vi "hydrolysis_reactor_setup.vi"(10 "#":i32) -> (2 "spec_file":path)   [LabVIEW 2019]
uses:
  lib/libSimulationControl/libSimulationControl.lvlib
  lib/libCheckpointUpdate/libCheckpointUpdate.lvlib
  lib/libFileFunctions/libFileFunctions.lvlib
panel:
  out "inflow path":path
  # "*******************************************************************\nBiogas Plant Control\n\nAuthor: Paul Zügel\nGCSC-Frankfurt am Main 2020\n\n*******************************************************************"
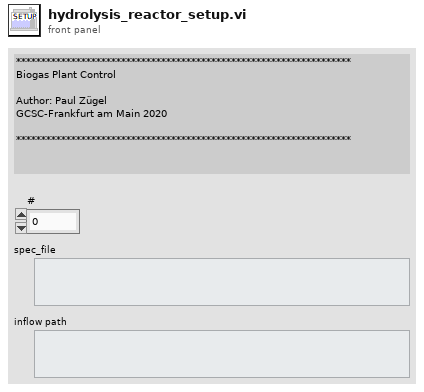
[diagram p1: front panel]
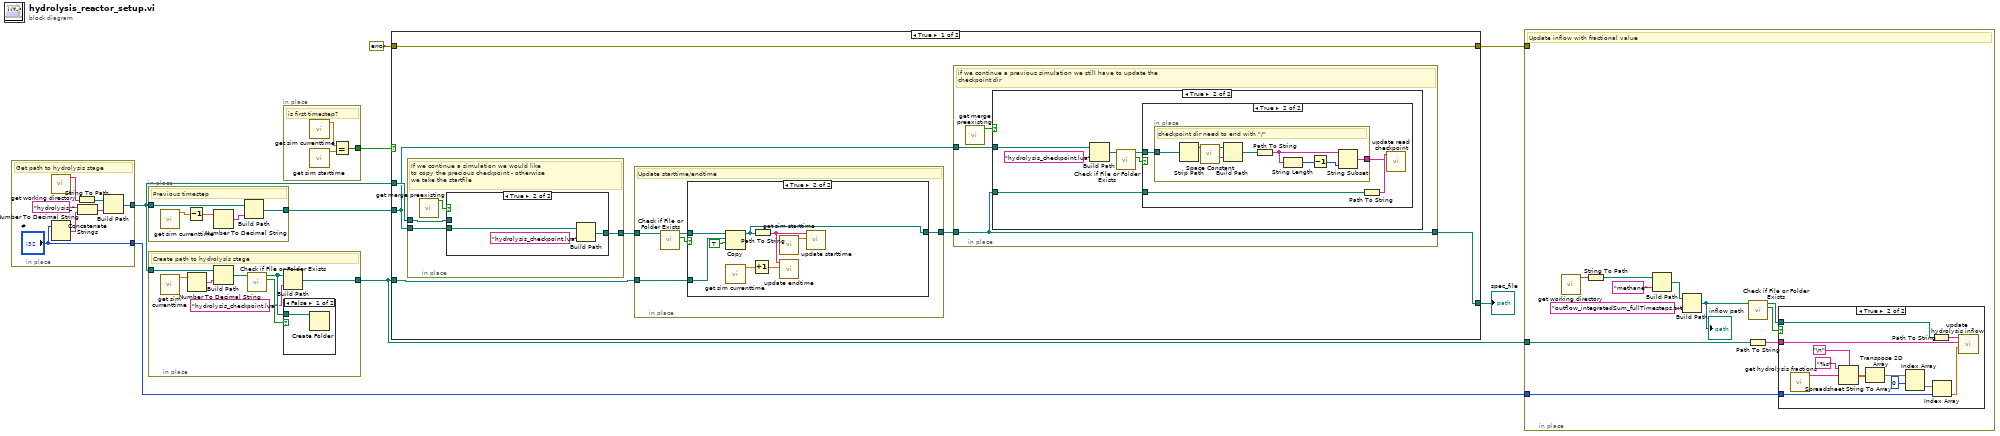
[diagram p0: block diagram]
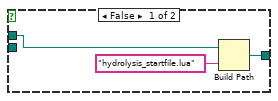
[diagram p4: hidden frame]
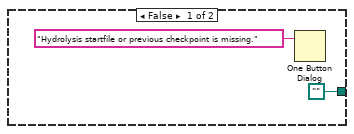
[diagram p5: hidden frame]
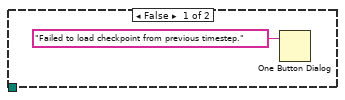
[diagram p7: hidden frame]
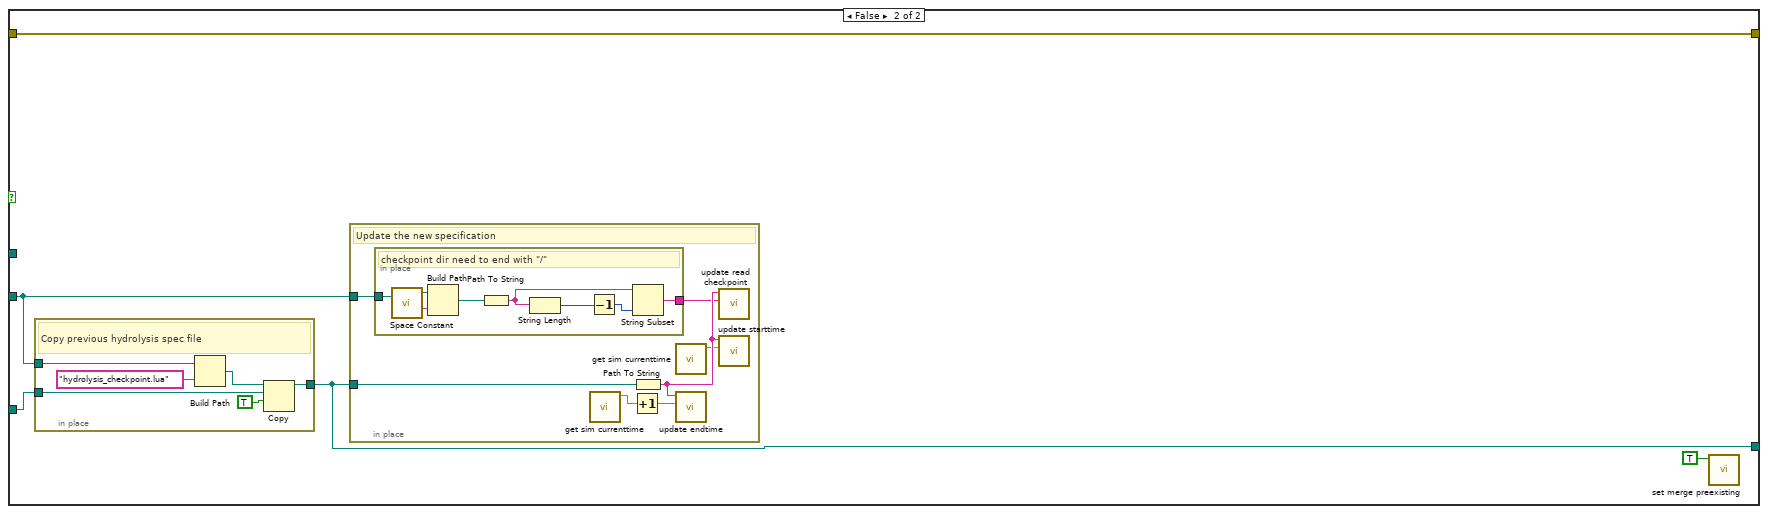
[diagram p8: hidden frame]
diagram:
  n1 = in-place {
    in-place-border: [w10] -> w4
    in-place-border: ["#"] -> w3
    # "Get path to hydrolysis stage"
    n2 = call "get working directory.vi"() -> ("function return"=w14:string)  [unwired: 10 in, 1 out]
    n3 = Number To Decimal String(number="#") -> (decimal integer string=w15:string)  [unwired: 1 in]
    n4 = String To Path(string=w14) -> (path=w11:path)
    n5 = Concatenate Strings("hydrolysis_" ("string"), w15) -> (w13:string)
    n6 = Build Path(base path=w11, name or relative path=w13) -> (appended path=w10:path)
  }
  n7 = in-place {
    in-place-border: [w18] -> w5
    in-place-border: w4 -> [w16]
    # "Previous timestep"
    n8 = call "get sim currenttime.vi"() -> ("current_time"=w17:dbl)  [unwired: 10 in, 1 out]
    n9 = Decrement(x=w17) -> (x-1=w20:dbl)
    n10 = Number To Decimal String(number=w20) -> (decimal integer string=w19:string)  [unwired: 1 in]
    n11 = Build Path(base path=w16, name or relative path=w19) -> (appended path=w18:path)
  }
  n12 = in-place {
    in-place-border: [w23] -> w7
    in-place-border: w4 -> [w21]
    # "Create path to hydrolysis stage"
    n13 = call "get sim currenttime.vi"() -> ("current_time"=w22:dbl)  [unwired: 10 in, 1 out]
    n14 = Number To Decimal String(number=w22) -> (decimal integer string=w27:string)  [unwired: 1 in]
    n15 = Build Path(base path=w21, name or relative path=w27) -> (appended path=w26:path)
    n16 = call <vilib>:"Check if File or Folder Exists.vi"("path"=w26) -> ("file or folder exists?"=w28:bool, "dup path"=w25:path)  [unwired: 8 in, 1 out]
    n17 = Build Path(base path=w25, name or relative path="hydrolysis_checkpoint.lua" ("string")) -> (appended path=w23:path)
    n18 = case shown="False" w28 {
      tunnel: w25 -> [w29 _]
      frame False {
        n19 = Create Folder(path (use dialog)=w29) -> ()  [unwired: 2 in, 3 out]
      }
      frame True {
      }
    }
  }
  n20 = in-place {
    in-place-border: [w32] -> w8
    # "is first timestep?"
    n21 = call "get sim currenttime.vi"() -> ("current_time"=w30:dbl)  [unwired: 10 in, 1 out]
    n22 = call "get sim starttime.vi"() -> ("sim_starttime"=w31:dbl)  [unwired: 10 in, 1 out]
    n23 = Equal?(x=w30, y=w31) -> (x = y?=w32:bool)
  }
  n24 = case shown="True" w8 {
    tunnel: w7 -> [w35 w89]
    tunnel: [w39 w91] -> w6
    tunnel: w5 -> [w36 w90]
    tunnel: w4 -> [w37 _]
    tunnel: errorcluster {"status"=FALSE, "code"=0, "source"=""} ("error constant") -> [w33 w87]
    tunnel: [w33 w87] -> w1
    frame True {
      n25 = in-place {
        in-place-border: [w43] -> w38
        in-place-border: w37 -> [w41]
        in-place-border: w36 -> [w40]
        # "If we continue a simulation we would like\nto copy the precious checkpoint - otherwise\nwe take the startfile"
        n26 = call "get merge preexisting.vi"() -> ("function return"=w42:bool)  [unwired: 10 in, 1 out]
        n27 = case shown="True" w42 {
          tunnel: [w45 w48] -> w43
          tunnel: w41 -> [w44 _]
          tunnel: w40 -> [_ w47]
          frame False {
            # "Copy base specification and update starttime/endtime"
            n28 = Build Path(base path=w44, name or relative path="hydrolysis_startfile.lua") -> (appended path=w45:path)
          }
          frame True {
            # "Copy previous hydrolysis spec file"
            n29 = Build Path(base path=w47, name or relative path="hydrolysis_checkpoint.lua" ("string")) -> (appended path=w48:path)
          }
        }
      }
      n30 = in-place {
        in-place-border: w38 -> [w52]
        in-place-border: w35 -> [w51]
        in-place-border: [w50] -> w34
        # "Update starttime/endtime"
        n31 = call <vilib>:"Check if File or Folder Exists.vi"("path"=w52) -> ("file or folder exists?"=w53:bool, "dup path"=w54:path)  [unwired: 8 in, 1 out]
        n32 = case shown="True" w53 {
          tunnel: [path "" w64] -> w50
          tunnel: w54 -> [_ w61]
          tunnel: w51 -> [_ w60]
          frame False {
            n33 = One Button Dialog(message="Hydrolysis startfile or previous checkpoint is missing.") -> ()  [unwired: 1 in, 1 out]
          }
          frame True {
            # "Update starttime/endtime"
            n34 = Copy(9:TRUE ("overwrite (F)"), 10:w60, 11:w61) -> (3:w64:path)  [unwired: 2 in, 2 out]
            n35 = call "get sim currenttime.vi"() -> ("current_time"=w59:dbl)  [unwired: 10 in, 1 out]
            n36 = Increment(x=w59) -> (x+1=w58:dbl)
            n37 = Path To String(path=w64) -> (string=w62:string)
            n38 = call "get sim starttime.vi"() -> ("sim_starttime"=w57:dbl)  [unwired: 10 in, 1 out]
            n39 = call "update endtime.vi"("endtime"=w58, "spec_dir"=w62) -> ()  [unwired: 9 in, 1 out]
            n40 = call "update starttime.vi"("starttime"=w57, "spec_dir"=w62) -> ()  [unwired: 9 in, 1 out]
          }
        }
      }
      n41 = in-place {
        in-place-border: [w65] -> w39
        in-place-border: w36 -> [w66]
        in-place-border: w34 -> [w65]
        # "if we continue a previous simulation we still have to update the \ncheckpoint dir"
        n42 = call "get merge preexisting.vi"() -> ("function return"=w67:bool)  [unwired: 10 in, 1 out]
        n43 = case shown="True" w67 {
          tunnel: w66 -> [_ w72]
          tunnel: w65 -> [_ w68]
          frame False {
          }
          frame True {
            n44 = Build Path(base path=w72, name or relative path="hydrolysis_checkpoint.lua" ("string")) -> (appended path=w71:path)
            n45 = call <vilib>:"Check if File or Folder Exists.vi"("path"=w71) -> ("file or folder exists?"=w69:bool, "dup path"=w70:path)  [unwired: 8 in, 1 out]
            n46 = case shown="True" w69 {
              tunnel: w70 -> [_ w76]
              tunnel: w68 -> [_ w77]
              frame False {
                n47 = One Button Dialog(message="Failed to load checkpoint from previous timestep.") -> ()  [unwired: 1 in, 1 out]
              }
              frame True {
                n48 = in-place {
                  in-place-border: w76 -> [w86]
                  in-place-border: [w79] -> w75
                  # "checkpoint dir need to end with \"/\""
                  n49 = Strip Path(path=w86) -> (stripped path=w80:path)  [unwired: 1 out]
                  n50 = call <vilib>:"Space Constant.vi"() -> ("String"=w81:string)
                  n51 = Build Path(base path=w80, name or relative path=w81) -> (appended path=w84:path)
                  n52 = Path To String(path=w84) -> (string=w85:string)
                  n53 = String Length(string=w85) -> (length=w83:i32)
                  n54 = Decrement(x=w83) -> (x-1=w82:i32)
                  n55 = String Subset(string=w85, length (rest)=w82) -> (substring=w79:string)  [unwired: 1 in]
                }
                n56 = Path To String(path=w77) -> (string=w78:string)
                n57 = call "update read checkpoint.vi"("checkpoint_dir"=w75, "spec_dir"=w78) -> ()  [unwired: 9 in, 1 out]
              }
            }
          }
        }
      }
    }
    frame False {
      n58 = in-place {
        in-place-border: w89 -> [w108]
        in-place-border: [w107] -> w91
        in-place-border: w90 -> [w106]
        # "Copy previous hydrolysis spec file"
        n59 = Build Path(base path=w106, name or relative path="hydrolysis_checkpoint.lua" ("string")) -> (appended path=w110:path)
        n60 = Copy(9:TRUE ("overwrite (F)"), 10:w108, 11:w110) -> (3:w107:path)  [unwired: 2 in, 2 out]
      }
      n61 = in-place {
        in-place-border: w90 -> [w92]
        in-place-border: w91 -> [w94]
        # "Update the new specification"
        n62 = in-place {
          in-place-border: [w100] -> w93
          in-place-border: w92 -> [w99]
          # "checkpoint dir need to end with \"/\""
          n63 = call <vilib>:"Space Constant.vi"() -> ("String"=w101:string)
          n64 = Build Path(base path=w99, name or relative path=w101) -> (appended path=w104:path)
          n65 = Path To String(path=w104) -> (string=w105:string)
          n66 = String Length(string=w105) -> (length=w103:i32)
          n67 = Decrement(x=w103) -> (x-1=w102:i32)
          n68 = String Subset(string=w105, length (rest)=w102) -> (substring=w100:string)  [unwired: 1 in]
        }
        n69 = call "get sim currenttime.vi"() -> ("current_time"=w96:dbl)  [unwired: 10 in, 1 out]
        n70 = Increment(x=w96) -> (x+1=w95:dbl)
        n71 = Path To String(path=w94) -> (string=w98:string)
        n72 = call "get sim currenttime.vi"() -> ("current_time"=w97:dbl)  [unwired: 10 in, 1 out]
        n73 = call "update endtime.vi"("endtime"=w95, "spec_dir"=w98) -> ()  [unwired: 9 in, 1 out]
        n74 = call "update read checkpoint.vi"("checkpoint_dir"=w93, "spec_dir"=w98) -> ()  [unwired: 9 in, 1 out]
        n75 = call "update starttime.vi"("starttime"=w97, "spec_dir"=w98) -> ()  [unwired: 9 in, 1 out]
      }
      n76 = call "set merge preexisting.vi"("merge"=TRUE) -> ()  [unwired: 10 in, 1 out]
    }
  }
  "spec_file" <- w6
  n77 = in-place "In Place Element Structure" {
    in-place-border: w7 -> [w114]
    in-place-border: w3 -> [w112]
    in-place-border: w1 -> [_]
    # "Update inflow with fractional value"
    n78 = call "get working directory.vi"() -> ("function return"=w122:string)  [unwired: 10 in, 1 out]
    n79 = String To Path(string=w122) -> (path=w121:path)
    n80 = Build Path(base path=w121, name or relative path="methane") -> (appended path=w119:path)
    n81 = Build Path(base path=w119, name or relative path="outflow_integratedSum_fullTimesteps.txt") -> (appended path=w117:path)
    "inflow path" <- w117
    n82 = Path To String(path=w114) -> (string=w113:string)
    n83 = call <vilib>:"Check if File or Folder Exists.vi"("path"=w117) -> ("file or folder exists?"=w116:bool, "dup path"=w115:path)  [unwired: 8 in, 1 out]
    n84 = case shown="True" w116 {
      tunnel: w115 -> [_ w134]
      tunnel: w113 -> [_ w133]
      tunnel: w112 -> [_ w124]
      frame False {
      }
      frame True {
        n85 = call "get hydrolysis fractions.vi"() -> ("function return"=w131:string)  [unwired: 10 in, 1 out]
        n86 = Spreadsheet String To Array(delimiter (Tab)="\n", format string="%s", spreadsheet string=w131) -> (array=w129:dbl[][])  [unwired: 1 in]
        n87 = Transpose 2D Array(2D array=w129) -> (transposed array=w130:dbl[][])
        n88 = Index Array(array=w130, index (row)=0) -> (element=w125:dbl[])  [unwired: 1 in]
        n89 = Path To String(path=w134) -> (string=w132:string)
        n90 = Index Array(array=w125, index=w124) -> (element=w123:dbl)
        n91 = call "update hydrolysis inflow.vi"("fraction"=w123, "hydrolysis_specfiles"=w133, "outflow_infile"=w132) -> ()  [unwired: 8 in, 1 out]
      }
    }
  }
